vi "cmd_multi.vi"(4 "chan_lower limit":i32=1, 5 "value format":string="%#.8g", 6 "chan_upper limit":i32=2, 7 "template":string="SOUR<channel>:VOLT:LOW <value>", 9 "scale_channels":dbl[](array[numeric])=[1.0, 1.0] format="%#_13f", 10 "channel_list":string="1, 2", 11 "value":dbl format="%#.8g") -> (2 "cmds":string[](array[string]), 3 "channel_array":i32[](array[numeric]))   [LabVIEW 2017, in "serial.lvlib"]
uses:
  serial.lvlib
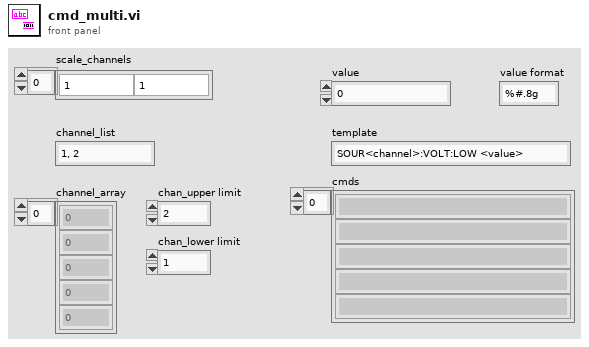
[diagram p1: front panel]
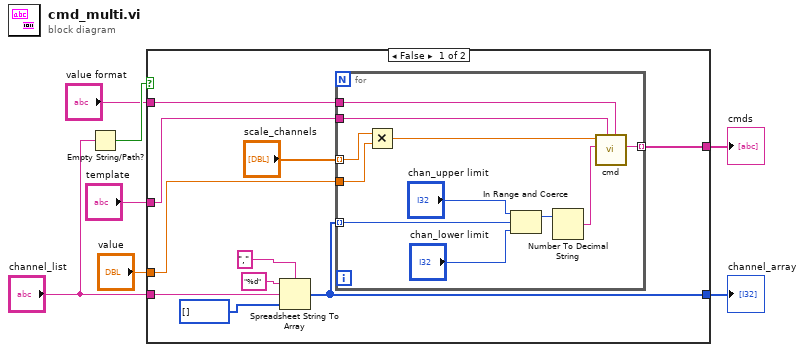
[diagram p0: block diagram]
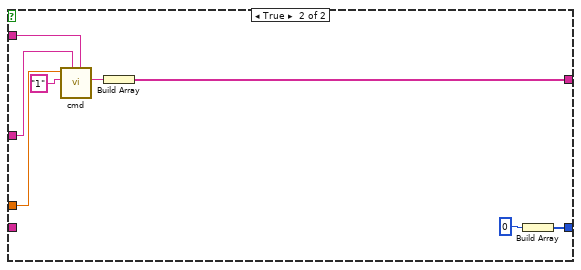
[diagram p2: hidden frame]
diagram:
  n1 = Empty String/Path?(string/path="channel_list") -> (empty?=w3:bool)
  n2 = case shown="False" w3 {
    tunnel: [w14 w30] -> w7
    tunnel: "value" -> [w13 w35]
    tunnel: [w12 w31] -> w5
    tunnel: "channel_list" -> [w11 _]
    tunnel: "value format" -> [w10 w33]
    tunnel: "template" -> [w9 w34]
    frame False {
      n3 = Spreadsheet String To Array(delimiter (Tab)=",", format string="%d", spreadsheet string=w11, array type (2D Dbl)=i32[] []) -> (array=w14:i32[])
      n4 = for {
        tunnel: w14 -> [w28] mode=indexing
        tunnel: w13 -> [w19]
        tunnel: [w21] -> w12 mode=indexing
        tunnel: w10 -> [w23]
        tunnel: w9 -> [w24]
        tunnel: "scale_channels" -> [w20] mode=indexing
        n5 = Multiply(x=w20, y=w19) -> (x*y=w18:dbl)
        n6 = In Range and Coerce(upper limit="chan_upper limit", x=w28, lower limit="chan_lower limit") -> (coerced(x)=w25:i32)  [unwired: 1 out]
        n7 = Number To Decimal String(number=w25) -> (decimal integer string=w22:string)  [unwired: 1 in]
        n8 = call "cmd.vi"("value format"=w23, "template"=w24, "channel"=w22, "value"=w18) -> ("cmd"=w21:string)  [unwired: 7 in]
      }
    }
    frame True {
      n9 = call "cmd.vi"("value format"=w33, "template"=w34, "channel"="1" ("option"), "value"=w35) -> ("cmd"=w32:string)  [unwired: 7 in]
      n10 = Build Array(w32) -> (w31:string[])
      n11 = Build Array(0 ("element")) -> (w30:i32[])
    }
  }
  "channel_array" <- w7
  "cmds" <- w5
